vi "Check Status.vi"(8 "error in":errorcluster, 11 "GOLPI ref. in":T1={"pipe handle"={"lv_proc.dll file path"=path "", "process instance handle"=[], "debug mode"=FALSE, "debug data"=[]}, "fast read timeout [ms]"=500, "fast read settle time [ms]"=10, "fast read to multiple [ms]"=1, "max elements per input line"=100, "slow read timeout [ms]"=5000, "stdin double format specifier"="", "max elements per stdout output column"=100, "console mode bitstream"=FALSE, "bitstream first read timeout [ms]"=1000, "bitstream read timeout [ms]"=50, "struct transfer possible"=FALSE, "matlab mode"=FALSE}) -> (0 "error out":errorcluster, 2 "exited?":bool, 3 "GOLPI ref. out":T1={"pipe handle"={"lv_proc.dll file path"=path "", "process instance handle"=[], "debug mode"=FALSE, "debug data"=[]}, "fast read timeout [ms]"=500, "fast read settle time [ms]"=10, "fast read to multiple [ms]"=1, "max elements per input line"=100, "slow read timeout [ms]"=5000, "stdin double format specifier"="", "max elements per stdout output column"=100, "console mode bitstream"=FALSE, "bitstream first read timeout [ms]"=1000, "bitstream read timeout [ms]"=50, "struct transfer possible"=FALSE, "matlab mode"=FALSE})   [LabVIEW 2020, in "GOLPI library.lvlib"]
doc: "Check if GNU Octave is still running or the process exited.\n\n---\nGOLPI works only with lv_proc.dll library, which is part of vipm package or should be delivered together with packed library. Placement of this dll is selected in terminal of Start GNU Octave.vi."
uses:
  GOLPI library.lvlib
  GOLPI reference Type Def.ctl
  Pipe Handle.ctl
  LV Process library.lvlib
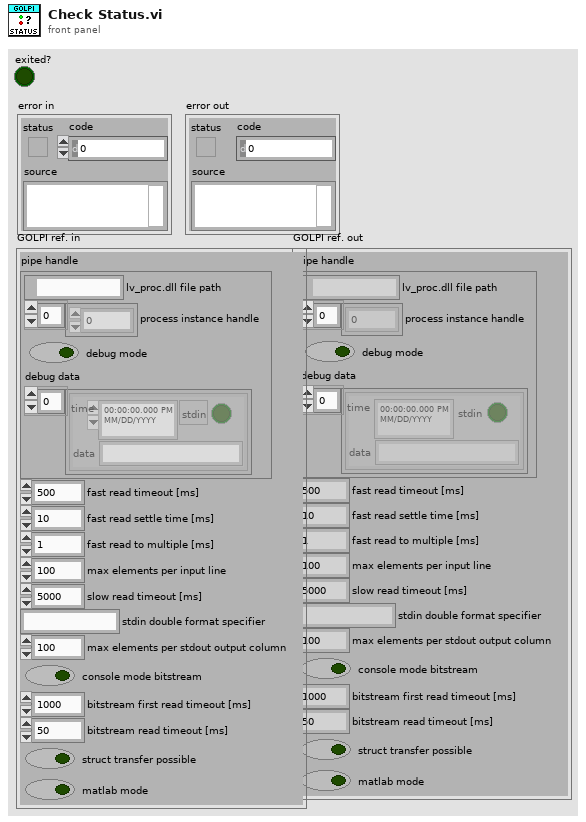
[diagram p1: front panel]
types:
  T1 = typedef "GOLPI library.lvlib/GOLPI reference Type Def.ctl" = cluster{"pipe handle":T2, "fast read timeout [ms]":u32, "fast read settle time [ms]":u32, "fast read to multiple [ms]":u32, "max elements per input line":u32, "slow read timeout [ms]":u32, "stdin double format specifier":string, "max elements per stdout output column":u32, "console mode bitstream":bool, "bitstream first read timeout [ms]":u32, "bitstream read timeout [ms]":u32, "struct transfer possible":bool, "matlab mode":bool}
  T2 = typedef "LV Process library.lvlib/Pipe Handle.ctl" = cluster{"lv_proc.dll file path":path, "process instance handle":u32[], "debug mode":bool, "debug data":cluster{"time":timestamp, "stdin":bool, "data":string}[]}
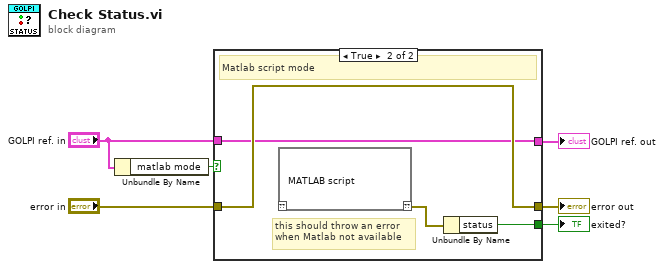
[diagram p0: block diagram]
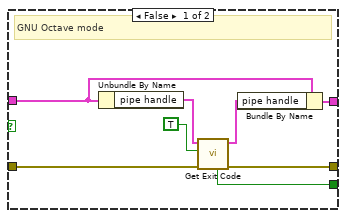
[diagram p2: hidden frame]
diagram:
  n1 = Unbundle By Name("GOLPI ref. in") -> ("matlab mode"=w2:bool)
  n2 = case shown="True" w2 {
    tunnel: "GOLPI ref. in" -> [w14 w15]
    tunnel: [w13 w15] -> w6
    tunnel: "error in" -> [w12 w18]
    tunnel: [w11 w18] -> w1
    tunnel: [w7 w16] -> w4
    frame False {
      # "GNU Octave mode"
      n3 = Unbundle By Name(w14) -> ("pipe handle"=w10:T2)
      n4 = call "Get Exit Code.vi"("error in"=w12, "ignore error if process running (T)"=TRUE ("ignore error if still active (T)"), "pipe in"=w10) -> ("error out"=w11:errorcluster, "pipe out"=w9:T2, "exited?"=w7:bool)  [unwired: 4 in, 2 out]
      n5 = Bundle By Name(cluster=w14, "pipe handle"=w9) -> (w13:T1)
    }
    frame True {
      # "this should throw an error\nwhen Matlab not available"
      # "Matlab script mode"
      n6 = script code="MATLAB script"() -> ("??"=w17:errorcluster)  [unwired: 1 in]
      n7 = Unbundle By Name(w17) -> ("status"=w16:bool)
    }
  }
  "error out" <- w1
  "GOLPI ref. out" <- w6
  "exited?" <- w4
